vi "MPM_Get_Range.vi"(8 "error in (no error)":errorcluster, 11 ".NET Reference in":refnum<k24>) -> (0 "error out":errorcluster, 2 "range out":i32, 3 "Reference out":refnum<k24>)   [LabVIEW 2017]
doc: "// -----get setting range for all slot"
uses:
  D:/test/FULLband-sts/Fullband_Sample/DLL/InstrumentDLL.dll
  DLL/InstrumentDLL.dll
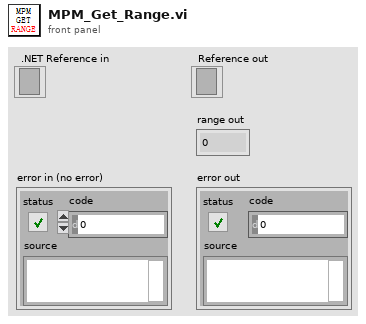
[diagram p1: front panel]
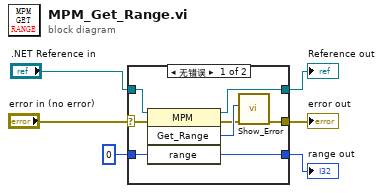
[diagram p0: block diagram]
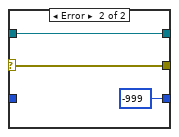
[diagram p2: hidden frame]
diagram:
  n1 = case shown="无错误" "error in (no error)" {
    selector: "error in (no error)" -> [w10 w15]
    tunnel: [w14 -999 ("range")] -> w6
    tunnel: [w13 w16] -> w5
    tunnel: ".NET Reference in" -> [w12 w16]
    tunnel: 0 ("range") -> [w11 _]
    tunnel: [w7 w15] -> w1
    frame No Error {
      n2 = invoke on="调用节点" class="MPM" method="Get_Range"(reference=w12, error in=w10, "range"=w11) -> (reference out=w13:refnum<k24>, error out=w8:errorcluster, "Get_Range"=w9:i32, "range"=w14:i32)  [unwired: 1 in]
      n3 = call "Show_Error.vi"("error in (no error)"=w8, "Error"=w9) -> ("error out"=w7:errorcluster)  [unwired: 9 in]
    }
    frame Error {
    }
  }
  "range out" <- w6
  "Reference out" <- w5
  "error out" <- w1
